vi "util-io-sort.vi"(10 "?":T1, 11 "IO Configs List":T2[](array[typedef]) {"calibration"."Y" format="%#.3f"; "calibration"."X" format="%#.3f"; "ADDR" format="%04d"}) -> (3 "Result":T2[](array[typedef]) {"calibration"."Y" format="%#.3f"; "calibration"."X" format="%#.3f"; "ADDR" format="%04d"})   [LabVIEW 2024]
uses:
  controls/IONode.ctl
  controls/type.address.ctl
  controls/enum.io.type.ctl
  controls/enum.io.mode.ctl
  controls/typeXyPoint.ctl
  controls/enum-io-sort-type.ctl
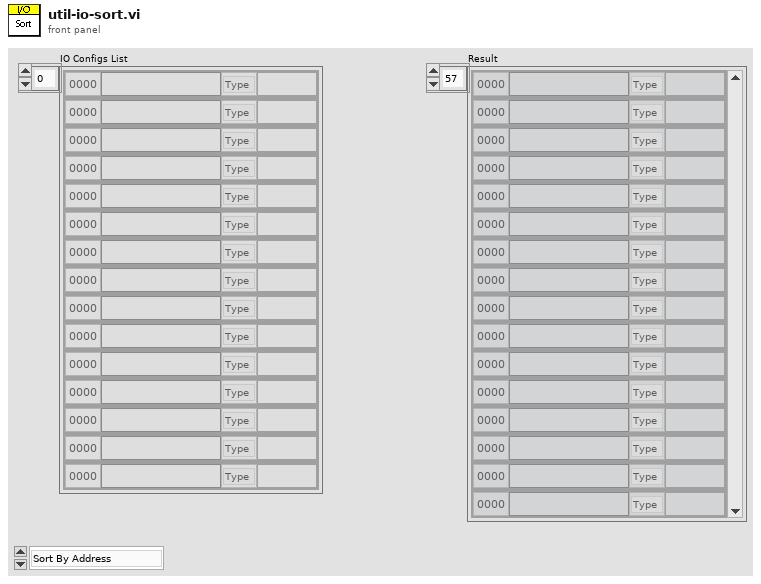
[diagram p1: front panel]
types:
  T1 = typedef "enum-io-sort-type.ctl" = enum16{"Sort By Address", "Sort By Name"}
  T2 = typedef "IONode.ctl" = cluster{"ADDR":T3, "Label":string, "Type":T4, "Mode":T5, "Value":string, "Tags":string, "calibration":T6[]}
  T3 = typedef "type.address.ctl" = u16
  T4 = typedef "enum.io.type.ctl" = enum16{"Type", "DI", "DO", "AI", "AO", "VL", "BUF"}
  T5 = typedef "enum.io.mode.ctl" = enum16{"Mode", "RIO", "SIM"}
  T6 = typedef "typeXyPoint.ctl" = cluster{"X":dbl, "Y":dbl}
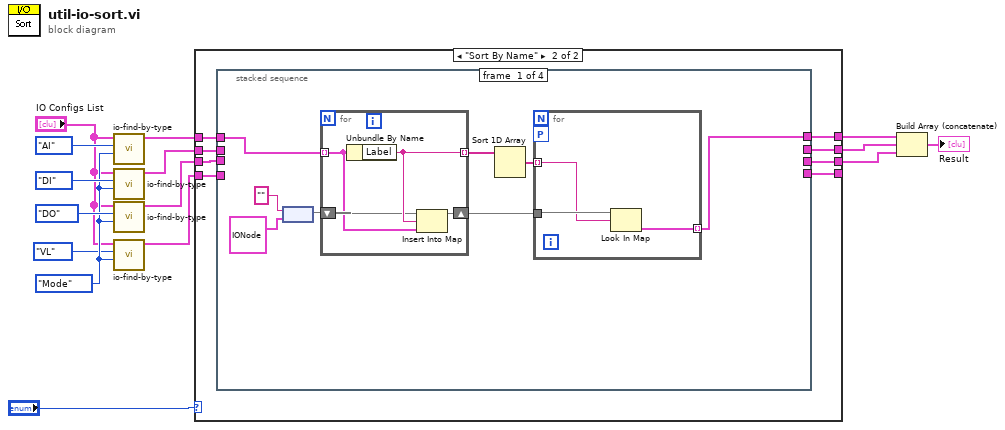
[diagram p0: block diagram]
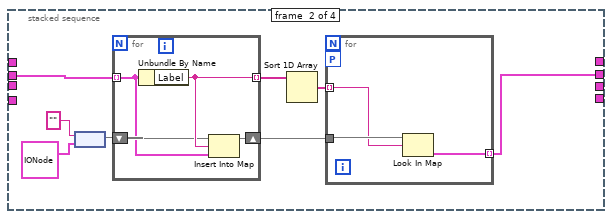
[diagram p3: hidden frame]
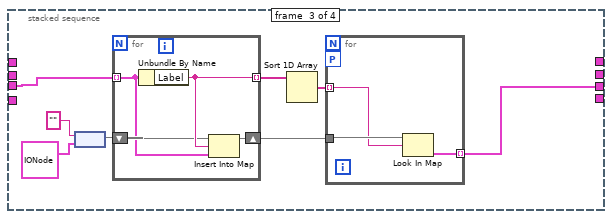
[diagram p4: hidden frame]
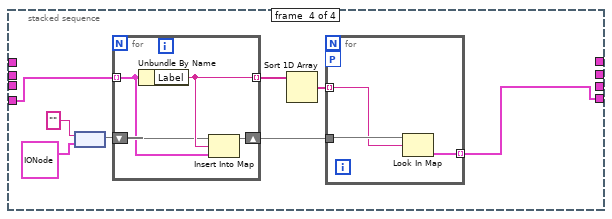
[diagram p5: hidden frame]
diagram:
  w4 = enum.io.mode."Mode" ("Mode(Any)")
  n1 = call "io-find-by-type.vi"("Mode(Any)"=w4, "Type"=enum.io.type."AI" ("type"), "IOConfigs in"="IO Configs List") -> ("Search Results"=w6:T2[])  [unwired: 8 in]
  n2 = call "io-find-by-type.vi"("Mode(Any)"=w4, "Type"=enum.io.type."DI" ("type"), "IOConfigs in"="IO Configs List") -> ("Search Results"=w10:T2[])  [unwired: 8 in]
  n3 = call "io-find-by-type.vi"("Mode(Any)"=w4, "Type"=enum.io.type."DO" ("type"), "IOConfigs in"="IO Configs List") -> ("Search Results"=w7:T2[])  [unwired: 8 in]
  n4 = call "io-find-by-type.vi"("Mode(Any)"=w4, "Type"=enum.io.type."VL", "IOConfigs in"="IO Configs List") -> ("Search Results"=w2:T2[])  [unwired: 8 in]
  n5 = case shown="\"Sort By Name\"" "?" {
    tunnel: w10 -> [w18 w27]
    tunnel: [w18 w26] -> w9
    tunnel: [w17 w25] -> w8
    tunnel: w7 -> [w17 w24]
    tunnel: w6 -> [w19 w23]
    tunnel: [w19 w22] -> w5
    tunnel: w2 -> [w16 w21]
    tunnel: [w16 w20] -> _
    frame "Sort By Address", Default {
    }
    frame "Sort By Name" {
      n6 = stacked-sequence {
        tunnel: w27 -> [_ w44 _ _]
        tunnel: [_ w43 _ _] -> w26
        tunnel: [_ _ w59 _] -> w25
        tunnel: w24 -> [_ _ w58 _]
        tunnel: w23 -> [w29 _ _ _]
        tunnel: [w28 _ _ _] -> w22
        tunnel: w21 -> [_ _ _ w73]
        tunnel: [_ _ _ w74] -> w20
        frame #0 {
          n7 = node("" ("key"), T2 {"ADDR"=0, "Label"="Name", "Type"=enum."DI", "Mode"=enum."RIO", "Value"="Value", "Tags"="Tags", "calibration"=[]} ("IoConf in 3")) -> (w31:map{string, T2})
          n8 = for {
            tunnel: w29 -> [w41] mode=indexing
            tunnel: [w42] -> w35 mode=indexing
            shift-right: [w40] -> w30
            shift-left: w31 -> [w39]
            n9 = Unbundle By Name(w41) -> ("Label"=w42:string)
            n10 = Insert Into Map(map in=w39, key=w42, value=w41) -> (map out=w40:map{string, T2})  [unwired: 2 out]
          }
          n11 = Sort 1D Array(array=w35) -> (sorted array=w34:string[])
          n12 = for {
            tunnel: w34 -> [w37] mode=indexing
            tunnel: w30 -> [w38]
            tunnel: [w36] -> w28 mode=indexing
            workers-P: _ -> [_]
            n13 = Look In Map(map=w38, key=w37) -> (value=w36:T2)  [unwired: 1 in, 1 out]
          }
        }
        frame #1 {
          n14 = node("" ("key"), T2 {"ADDR"=0, "Label"="Name", "Type"=enum."DI", "Mode"=enum."RIO", "Value"="Value", "Tags"="Tags", "calibration"=[]} ("IoConf in 3")) -> (w46:map{string, T2})
          n15 = for {
            tunnel: w44 -> [w56] mode=indexing
            tunnel: [w57] -> w50 mode=indexing
            shift-right: [w55] -> w45
            shift-left: w46 -> [w54]
            n16 = Unbundle By Name(w56) -> ("Label"=w57:string)
            n17 = Insert Into Map(map in=w54, key=w57, value=w56) -> (map out=w55:map{string, T2})  [unwired: 2 out]
          }
          n18 = Sort 1D Array(array=w50) -> (sorted array=w49:string[])
          n19 = for {
            tunnel: w49 -> [w52] mode=indexing
            tunnel: w45 -> [w53]
            tunnel: [w51] -> w43 mode=indexing
            workers-P: _ -> [_]
            n20 = Look In Map(map=w53, key=w52) -> (value=w51:T2)  [unwired: 1 in, 1 out]
          }
        }
        frame #2 {
          n21 = node("" ("key"), T2 {"ADDR"=0, "Label"="Name", "Type"=enum."DI", "Mode"=enum."RIO", "Value"="Value", "Tags"="Tags", "calibration"=[]} ("IoConf in 3")) -> (w61:map{string, T2})
          n22 = for {
            tunnel: w58 -> [w71] mode=indexing
            tunnel: [w72] -> w65 mode=indexing
            shift-right: [w70] -> w60
            shift-left: w61 -> [w69]
            n23 = Unbundle By Name(w71) -> ("Label"=w72:string)
            n24 = Insert Into Map(map in=w69, key=w72, value=w71) -> (map out=w70:map{string, T2})  [unwired: 2 out]
          }
          n25 = Sort 1D Array(array=w65) -> (sorted array=w64:string[])
          n26 = for {
            tunnel: w64 -> [w67] mode=indexing
            tunnel: w60 -> [w68]
            tunnel: [w66] -> w59 mode=indexing
            workers-P: _ -> [_]
            n27 = Look In Map(map=w68, key=w67) -> (value=w66:T2)  [unwired: 1 in, 1 out]
          }
        }
        frame #3 {
          n28 = node("" ("key"), T2 {"ADDR"=0, "Label"="Name", "Type"=enum."DI", "Mode"=enum."RIO", "Value"="Value", "Tags"="Tags", "calibration"=[]} ("IoConf in 3")) -> (w76:map{string, T2})
          n29 = for {
            tunnel: w73 -> [w86] mode=indexing
            tunnel: [w87] -> w80 mode=indexing
            shift-right: [w85] -> w75
            shift-left: w76 -> [w84]
            n30 = Unbundle By Name(w86) -> ("Label"=w87:string)
            n31 = Insert Into Map(map in=w84, key=w87, value=w86) -> (map out=w85:map{string, T2})  [unwired: 2 out]
          }
          n32 = Sort 1D Array(array=w80) -> (sorted array=w79:string[])
          n33 = for {
            tunnel: w79 -> [w82] mode=indexing
            tunnel: w75 -> [w83]
            tunnel: [w81] -> w74 mode=indexing
            workers-P: _ -> [_]
            n34 = Look In Map(map=w83, key=w82) -> (value=w81:T2)  [unwired: 1 in, 1 out]
          }
        }
      }
    }
  }
  n35 = Build Array (concatenate)(w5, w9, w8) -> (→"Result":T2[])
